vi "Problem 1.vi"(11 "Upper Limit":i32=1000) -> (2 "Numbers":i32[](array[numeric]), 3 "sum":i32)   [LabVIEW 2013, in "Problem 1.lvlib"]
uses:
  Problem 1.lvlib
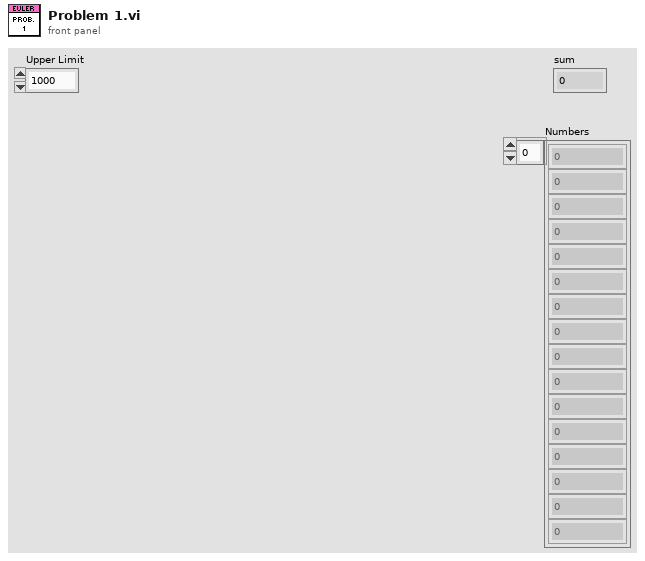
[diagram p1: front panel]
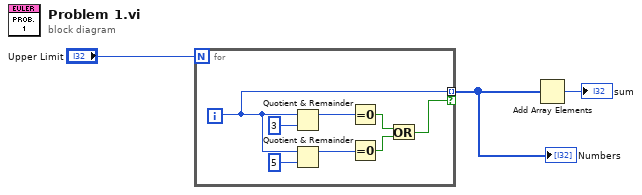
[diagram p0: block diagram]
diagram:
  n1 = for {
    N: "Upper Limit" -> [_]
    tunnel: [w5] -> w3 mode=indexing if=w4
    i -> [w5]
    n2 = Quotient & Remainder(x=w5, y=3) -> (x-y*floor(x/y)=w9:i32)  [unwired: 1 out]
    n3 = Quotient & Remainder(x=w5, y=5) -> (x-y*floor(x/y)=w8:i32)  [unwired: 1 out]
    n4 = Equal To 0?(x=w9) -> (x = 0?=w6:bool)
    n5 = Equal To 0?(x=w8) -> (x = 0?=w7:bool)
    n6 = Or(x=w6, y=w7) -> (x .or. y?=w4:bool)
  }
  "Numbers" <- w3
  n7 = Add Array Elements(numeric array=w3) -> (sum=→"sum":i32)
